vi "okDeviceSensors Get Sensor.vi"(8 "Error In":errorcluster, 9 "index":i32, 11 "okDeviceSensors Refnum":refnum<k24>) -> (0 "Error Out":errorcluster, 1 "okDeviceSensor":T1, 3 "okDeviceSensors Refnum":refnum<k24>)   [LabVIEW 2021, in "okFrontPanelC#Wrapper.lvlib"]
uses:
  okFrontPanelC#Wrapper.lvlib
  D:/UCLA Thinkpad Google Drive/LabVIEW 2021 SP1/builds/SwissSPAD Live Distribution/Opal Kelly/C# Wrapper/v5.0.2/libFrontPanel-csharp.dll
  v5.0.2/libFrontPanel-csharp.dll
  okDeviceSensor.ctl
  okDeviceSensorType.ctl
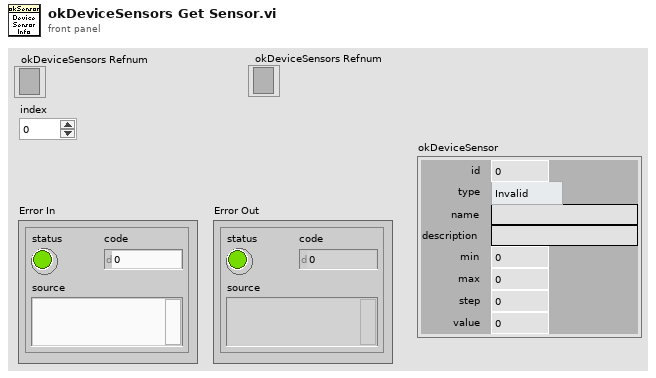
[diagram p1: front panel]
types:
  T1 = typedef "okFrontPanelC#Wrapper.lvlib/okDeviceSensor.ctl" = cluster{"id":i32, "type":T2, "name":string, "description":string, "min":dbl, "max":dbl, "step":dbl, "value":dbl}
  T2 = typedef "okFrontPanelC#Wrapper.lvlib/okDeviceSensorType.ctl" = enum16{"Invalid", "Boolean", "Integer", "Float", "Voltage", "Current", "Temperature", "Fan RPM"}
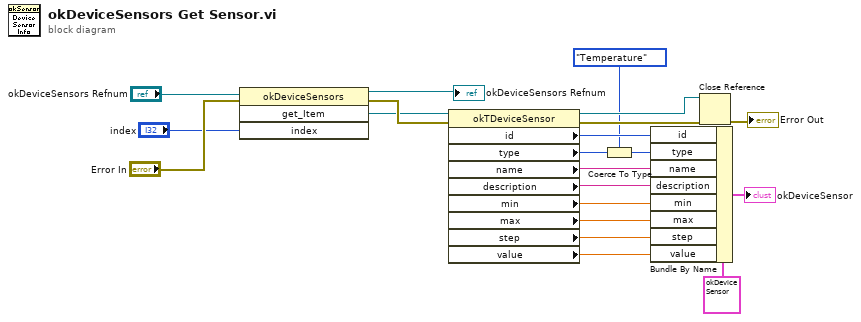
[diagram p0: block diagram]
diagram:
  n1 = invoke class="okDeviceSensors" method="get_Item"(reference="okDeviceSensors Refnum", error in="Error In", "index"="index") -> (reference out=→"okDeviceSensors Refnum":refnum<k24>, error out=w17:errorcluster, "get_Item"=w16:refnum<k24>)  [unwired: 1 in, 1 out]
  n2 = property class="okTDeviceSensor"(reference=w16, error in=w17) -> (reference out=w4:refnum<k24>, error out=w5:errorcluster, "id"=w15:i32, "type"=w14:i32, "name"=w13:string, "description"=w12:string, "min"=w11:dbl, "max"=w10:dbl, "step"=w9:dbl, "value"=w8:dbl)
  n3 = Coerce To Type(0:w14, 1:okDeviceSensorType."Temperature" ("type")) -> (2:w2:T2)
  n4 = Bundle By Name(cluster=T1 {"id"=0, "type"=enum."Invalid", "name"="", "description"="", "min"=0.0, "max"=0.0, "step"=0.0, "value"=0.0} ("okDeviceSensor"), "id"=w15, "type"=w2, "name"=w13, "description"=w12, "min"=w11, "max"=w10, "step"=w9, "value"=w8) -> (→"okDeviceSensor":T1)
  n5 = Close Reference(reference=w4, error in (no error)=w5) -> (error out=→"Error Out":errorcluster)
